vi "Self.vi"(9 "Is Priority":bool, 10 "Msg":refnum<class "Msg.lvclass">, 11 "Base Actor in":refnum<class "Base Actor.lvclass">) -> (3 "Base Actor out":refnum<class "Base Actor.lvclass">)   [LabVIEW 2020, in "jettl.lvlib" / "Actor.lvlib" / "Base Actor.lvclass"]
uses:
  Base Actor.lvclass
  Sender/Relation.ctl
  Sender/Sender.lvlib
  Msg/Msg.lvclass
  Error/Error.lvlib
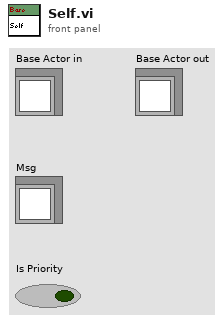
[diagram p1: front panel]
types:
  T1 = typedef "jettl.lvlib/Actor.lvlib/Implemented Msgs.ctl" = set{refnum<class "Msg.lvclass">}
  T2 = typedef "jettl.lvlib/Sender.lvlib/Relation.ctl" = enum16{"Self", "Creator", "Created"}
  T3 = typedef "jettl.lvlib/Actor.lvlib/Attributes.ctl" = cluster{"Alias":string, "Address":refnum<user-event>, "Implemented Msgs":T1, "Path":path}
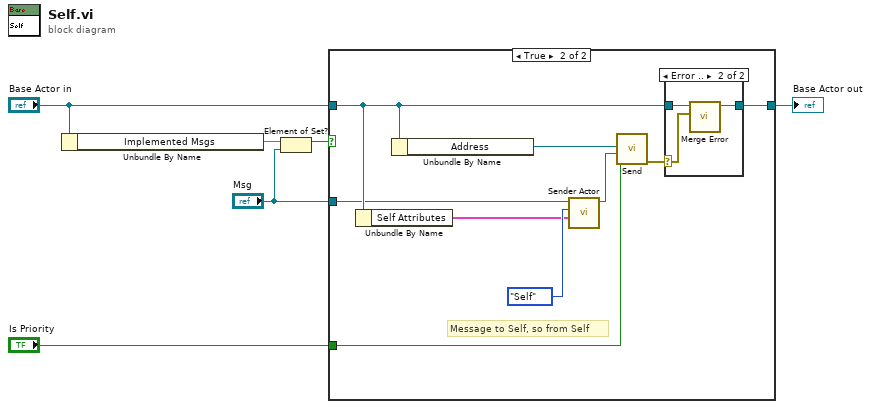
[diagram p0: block diagram]
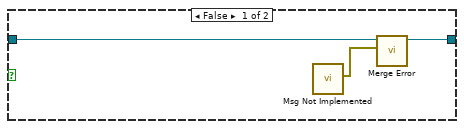
[diagram p2: hidden frame]
diagram:
  n1 = Unbundle By Name("Base Actor in") -> ("Implemented Msgs"=w3:T1)
  n2 = Element of Set?(10:"Msg", 11:w3) -> (3:w1:bool)
  n3 = case shown="True" w1 {
    tunnel: [w8 w18] -> w6
    tunnel: "Is Priority" -> [_ w17]
    tunnel: "Base Actor in" -> [w9 w13]
    tunnel: "Msg" -> [_ w12]
    frame False {
      n4 = call "Msg Not Implemented.vi"() -> ("Error"=w7:errorcluster)  [unwired: 11 in]
      n5 = call-dynamic "Merge Error.vi"("Error"=w7, "Base Actor in"=w9) -> ("Base Actor out"=w8:refnum<class "Base Actor.lvclass">)  [unwired: 9 in]
    }
    frame True {
      # "Message to Self, so from Self"
      n6 = Unbundle By Name(w13) -> ("Self Attributes"=w10:T3)
      n7 = Unbundle By Name(w13) -> ("Address"=w15:refnum<user-event>)
      n8 = call "Sender Actor.vi"("Self Attributes"=w10, "Relation"=Relation."Self", "Msg in"=w12) -> ("Msg out"=w14:refnum<class "Msg.lvclass">)  [unwired: 8 in]
      n9 = call "Send.vi"("Is Priority"=w17, "Msg"=w14, "Address"=w15) -> ("error out"=w16:errorcluster)  [unwired: 8 in]
      n10 = case shown="Error .." w16 {
        selector: w16 -> [_ w20]
        tunnel: [w19 w22] -> w18
        tunnel: w13 -> [w19 w21]
        frame No Error {
        }
        frame Error {
          n11 = call-dynamic "Merge Error.vi"("Error"=w20, "Base Actor in"=w21) -> ("Base Actor out"=w22:refnum<class "Base Actor.lvclass">)  [unwired: 9 in]
        }
      }
    }
  }
  "Base Actor out" <- w6
